vi "SIP_day03.vi"() -> ()   [LabVIEW 2025]
panel:
  in  "stop":bool
  out "string enum":string
  out "string selectt":string
  out "string case":string
  in  "Enum":enum16{"case1", "case2", "case3"}(ring)
  in  "Boolean":bool
  in  "q":bool
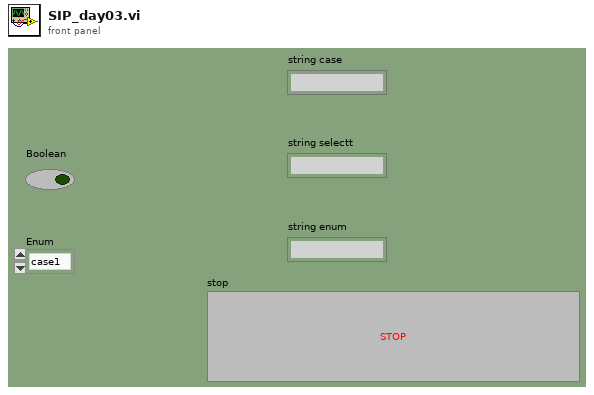
[diagram p1: front panel]
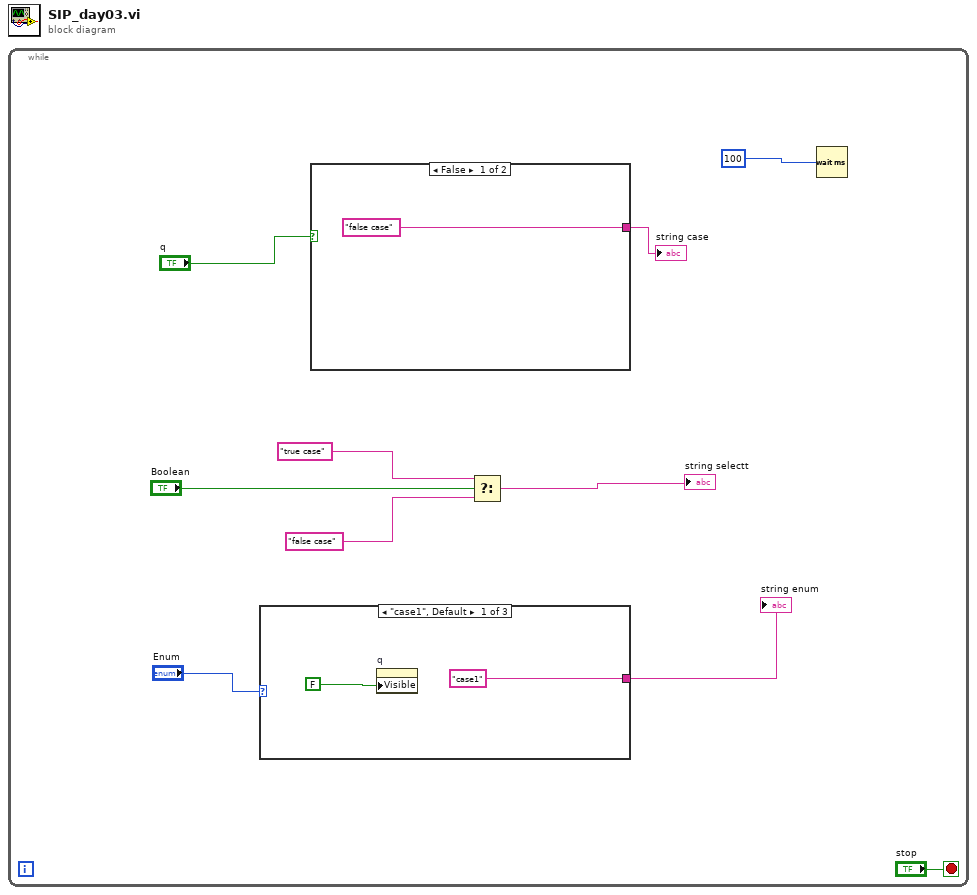
[diagram p0: block diagram]
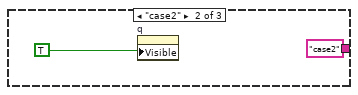
[diagram p2: hidden frame]
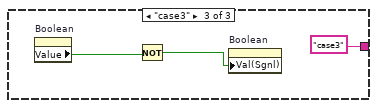
[diagram p3: hidden frame]
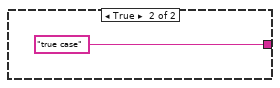
[diagram p4: hidden frame]
diagram:
  n1 = while {
    stop <- "stop" stop-if-true
    n2 = case shown="\"case1\", Default" "Enum" {
      tunnel: ["case1" "case2" "case3"] -> w3
      frame "case1", Default {
        n3 = property on="q" class="Bool (strict)"("Visible"=FALSE) -> ()  [unwired: 2 in, 2 out]
      }
      frame "case2" {
        n4 = property on="q" class="Bool (strict)"("Visible"=TRUE) -> ()  [unwired: 2 in, 2 out]
      }
      frame "case3" {
        n5 = property on="Boolean" class="Bool (strict)"() -> ("Value"=w15:bool)  [unwired: 2 in, 2 out]
        n6 = Not(x=w15) -> (.not. x?=w16:bool)
        n7 = property on="Boolean" class="Bool (strict)"("Val(Sgnl)"=w16) -> ()  [unwired: 2 in, 2 out]
      }
    }
    "string enum" <- w3
    n8 = case shown="False" "q" {
      tunnel: ["false case" "true case"] -> w9
      frame False {
      }
      frame True {
      }
    }
    "string case" <- w9
    n9 = Select(t="true case", s="Boolean", f="false case") -> (s? t:f=→"string selectt":string)
    n10 = Wait (ms)(milliseconds to wait=u32 100) -> ()  [unwired: 1 out]
  }
